vi "Store UID Data.vi"(6 "Assert Name":string, 7 "UID String":string, 8 "error in (no error)":errorcluster, 10 "Assert Count Value":i32, 11 "Standard Display Configuration in":refnum<class "Standard Display Configuration.lvclass">) -> (0 "error out":errorcluster, 3 "Standard Display Configuration out":refnum<class "Standard Display Configuration.lvclass">)   [LabVIEW 2018, in "Assert API Components.lvlib" / "Assert Display.lvlib" / "Main Display.lvlib" / "Standard Display Configuration.lvclass"]
doc: "Stores the UID index value in the variant data"
uses:
  Standard Display Configuration.lvclass
  C:/Users/UKHornP/Documents/Work/Projects/Assert_API/Core/Main Display/Display Configurations/Base Display Configuration.lvclass
  Base Display Configuration.lvclass/Base Display Configuration.ctl
  Base Display Configuration.lvclass
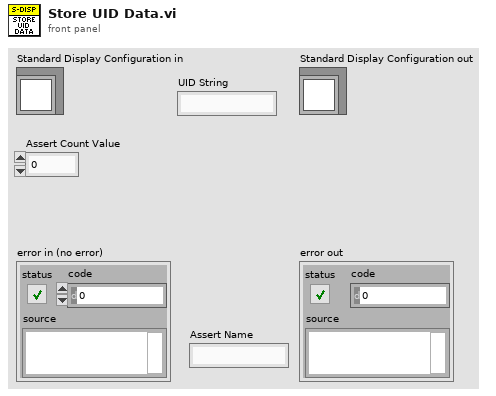
[diagram p1: front panel]
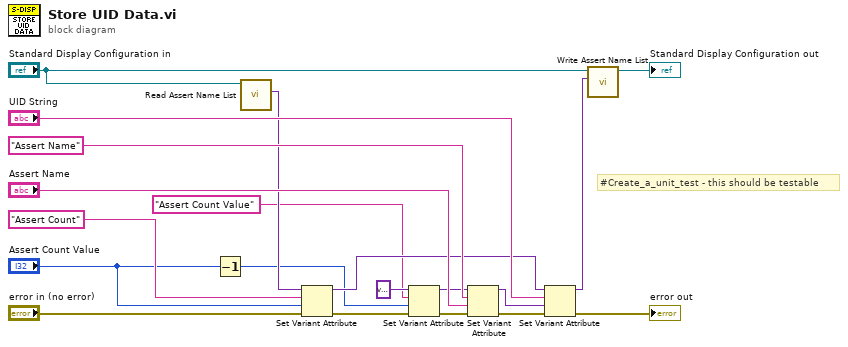
[diagram p0: block diagram]
diagram:
  # "#Create_a_unit_test - this should be testable"
  n1 = Decrement(x="Assert Count Value") -> (x-1=w1:i32)
  n2 = call "Read Assert Name List.vi"("Base Display Configuration in"="Standard Display Configuration in") -> ("Assert Name List"=w8:variant)  [unwired: 10 in]
  n3 = Set Variant Attribute(Variant=w8, name="Assert Count", value="Assert Count Value", error in="error in (no error)") -> (Variant out=w7:variant, error out=w14:errorcluster)  [unwired: 1 out]
  n4 = Set Variant Attribute(Variant=variant ("variant"), name="Assert Count Value", value=w1, error in=w14) -> (Variant out=w4:variant, error out=w6:errorcluster)  [unwired: 1 out]
  n5 = Set Variant Attribute(Variant=w4, name="Assert Name", value="Assert Name", error in=w6) -> (Variant out=w9:variant, error out=w13:errorcluster)  [unwired: 1 out]
  n6 = Set Variant Attribute(Variant=w7, name="UID String", value=w9, error in=w13) -> (Variant out=w18:variant, error out=→"error out":errorcluster)  [unwired: 1 out]
  n7 = call "Write Assert Name List.vi"("Assert Name List"=w18, "Base Display Configuration in"="Standard Display Configuration in") -> ("Base Display Configuration out"=→"Standard Display Configuration out":refnum<class "Standard Display Configuration.lvclass">)  [unwired: 9 in]
